vi "Datalog Aggregator.vi"(5 "LuaVIEW reference":T1) -> (15 "error out":errorcluster)   [LabVIEW 2012]
doc: "This plug-in is required by the \"datalogging\" runlevel. It sets up the buffer that aggregates data to be logged and periodically copies over the data from the in-memory tag buffers while applying logging algorithms."
uses:
  luaview/typedefs/t_LuaVIEW Reference.ctl
  typedefs/t_Datalog Aggregator States.ctl
  typedefs/t_DataLog Aggregate New Points Methods.ctl
  typedefs/t_DataLog Tag Info List Methods.ctl
  typedefs/t_DataLog Tag Buffers Methods.ctl
  luaview/typedefs/t_LuaVIEW Task State Methods.ctl
  typedefs/t_DataLog Aggregation Buffer Methods.ctl
  typedefs/t_DataLog Tag Hash Methods.ctl
  subvis/private/glb_DataLog Runtime Parameterisation.vi
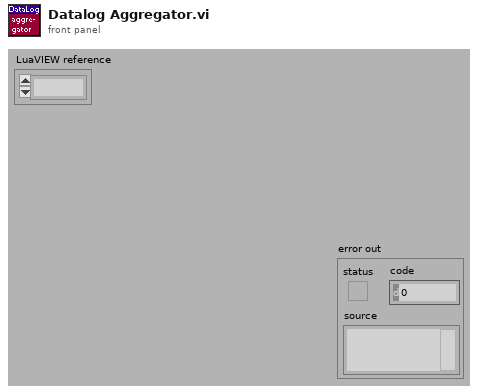
[diagram p1: front panel]
types:
  T1 = typedef "t_LuaVIEW Reference.ctl" = refnum<k1>
  T2 = typedef "t_Datalog Aggregator States.ctl" = enum16{"empty queue", "do aggregation", "undefine", "initialize", "init aggreg obj", "init undefine", "init active", "cleanup", "clean undefine", "clean buffers", "clean aggreg obj", "clean flush", "stop"}
  T3 = typedef "t_DataLog Aggregate New Points Methods.ctl" = enum16{"initialize", "aggregate", "cleanup"}
  T4 = typedef "t_DataLog Tag Info List Methods.ctl" = enum16{"initialize", "create", "create empty", "rename", "delete", "test tag", "get", "get by name", "get default", "get list", "get path", "get subsets", "set subsets", "set config", "set capacity", "#tags", "go live", "set unlocked", "set mirrored"}
  T5 = typedef "t_DataLog Tag Buffers Methods.ctl" = enum16{"initialize", "inert", "write", "read", "read oldest", "read last", "cleanup"}
  T6 = typedef "t_LuaVIEW Task State Methods.ctl" = enum16{"cleanup", "set initial", "set mode", "set active mode", "set error", "get task info", "get script info", "set signal", "clear signal", "test handled", "test delegated", "test signal", "handle signal", "delegate signal", "allow signal", "disallow signal", "disallow all", "signals?", "delegated signals?", "protection++", "protection--", "protection=0", "message", "next message", "pop message", "message available?", "force stop", "set swap preps", "apply swap preps"}
  T7 = typedef "t_DataLog Tag Hash Methods.ctl" = enum16{"initialize", "add tag", "index tag", "lookup", "#tags", "cleanup", "write recovery", "read recovery", "delete recovery"}
  T8 = typedef "t_DataLog Aggregation Buffer Methods.ctl" = enum16{"initialize", "write", "write special", "flush", "flush next", "flush next if", "setup recovery", "update recovery", "verify recovery", "dummy flush ", "cleanup"}
  T9 = typedef "t_DataLog Tag Config.ctl" = cluster{"name":string, "unit":string, "temporal":T10, "value":T11, "index":i32, "capacity":i32, "is meta?":bool, "mincapacity":i32, "deadband":dbl, "limit delay":dbl, "format":T12, "precision":u8, "undefine":bool, "update":bool, "update period":u16, "expression":string, "description":string, "logging algorithm":T13, "logging parameters":dbl[]}
  T10 = typedef "t_DataLog Temporal Types.ctl" = enum16{"set&hold", "sample", "event"}
  T11 = typedef "t_DataLog Value Types.ctl" = enum16{"number", "string"}
  T12 = typedef "t_DataLog Numerical Format.ctl" = enum8{"fractional", "exponential", "engineering"}
  T13 = typedef "t_DataLog Logging Algorithms.ctl" = enum16{"nothing", "changes", "everything", "every Nth", "time threshold", "value threshold + prior", "t or v threshold", "t or v threshold + prior"}
  T14 = typedef "t_DataLog Point.ctl" = cluster{"time":dbl, "value":dbl}
  T15 = typedef "t_LuaVIEW Task State Pane.ctl" = refnum<vi>
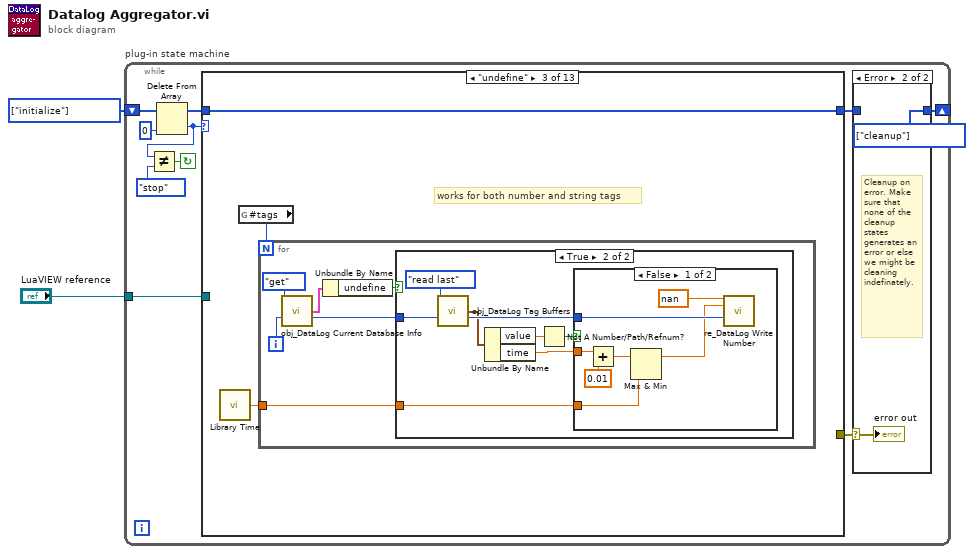
[diagram p0: block diagram]
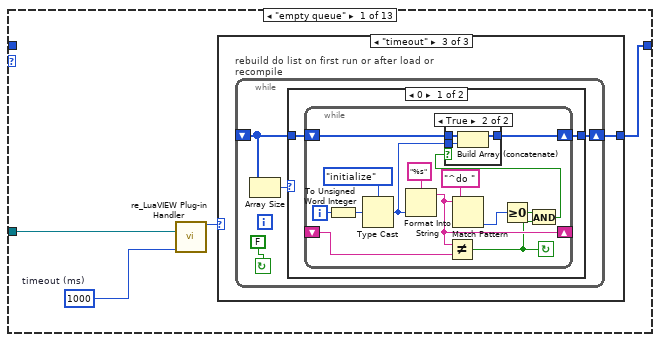
[diagram p3: hidden frame]
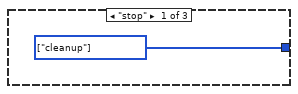
[diagram p4: hidden frame]
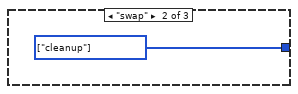
[diagram p5: hidden frame]
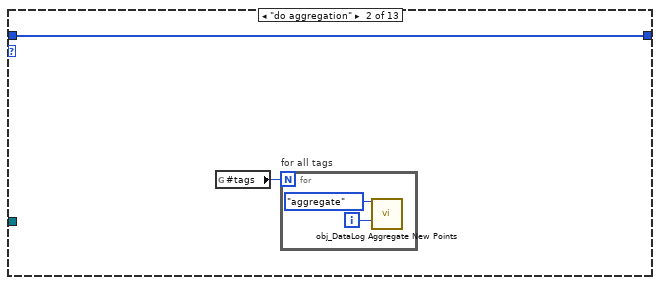
[diagram p8: hidden frame]
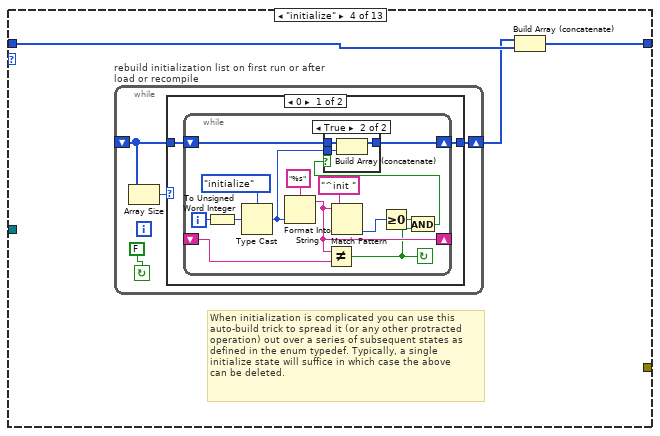
[diagram p11: hidden frame]
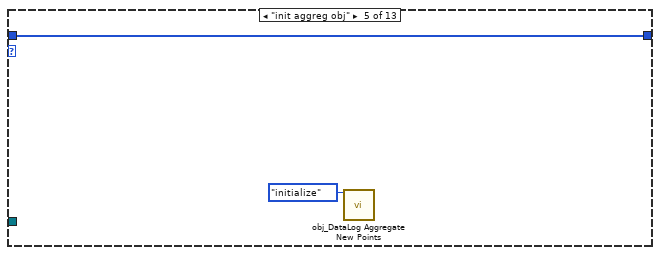
[diagram p14: hidden frame]
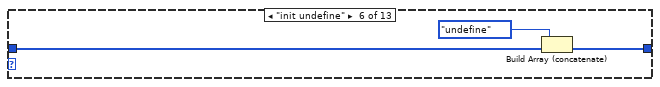
[diagram p15: hidden frame]
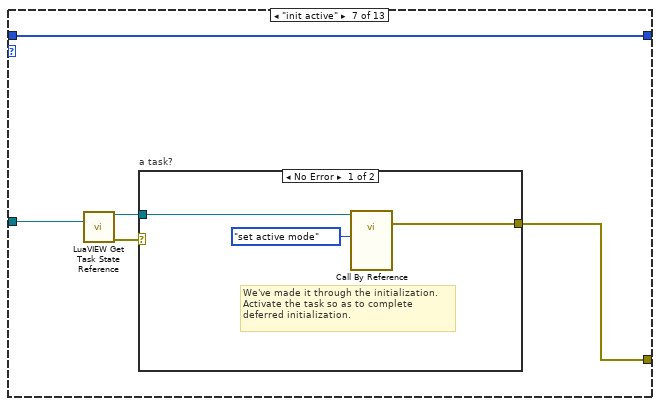
[diagram p16: hidden frame]
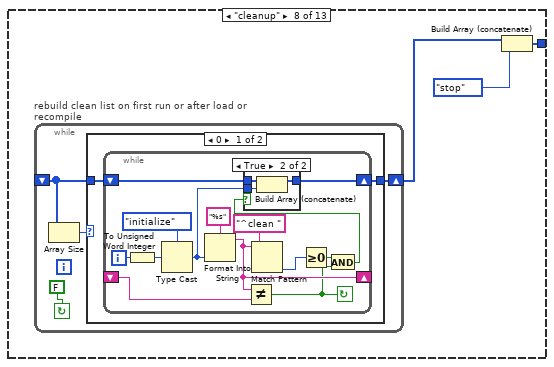
[diagram p18: hidden frame]
diagram:
  w2 = T2[] [enum."initialize"] items=["empty queue", "do aggregation", "undefine", "initialize", "init aggreg obj", "init undefine", "init active", "cleanup", "clean undefine", "clean buffers", "clean aggreg obj", "clean flush", "stop"] ("Array Constant")
  n1 = while "plug-in state machine" {
    shift-left: w2 -> [w10]
    shift-right: [w5] -> _
    tunnel: "LuaVIEW reference" -> [w7]
    stop <- w12 continue-if-true
    n2 = Delete From Array(array=w10, index=0) -> (deleted portion=w3:T2, array with subset deleted=w9:T2[])  [unwired: 1 in]
    n3 = Not Equal?(x=w3, y=t_Datalog_Aggregator_States."stop" ("states")) -> (x != y?=w12:bool)
    n4 = case "Case" shown="\"undefine\"" w3 {
      tunnel: [w19 w49 w54 w78 w105 w107 w113 w119 w146 w150 w152 w153 w159] -> w6
      tunnel: w9 -> [_ w49 w54 w77 w105 w108 w113 _ w147 w148 w152 w153 w159]
      tunnel: w7 -> [w17 _ _ _ _ _ w110 _ _ _ _ _ _]
      tunnel: [_ _ _ _ _ _ w112 _ _ _ _ _ _] -> w4
      frame "empty queue" {
        w16 = 1000  # timeout (ms)
        n5 = call "re_LuaVIEW Plug-in Handler.vi"("LuaVIEW reference"=w17, "timeout (ms)"=w16) -> ("handle"=w18:enum16{"timeout", "swap", "stop"})  [unwired: 13 in]
        n6 = case shown="\"timeout\"" w18 {
          tunnel: [w20 w21 w22] -> w19
          frame "stop" {
            w20 = T2[] [enum."cleanup"] items=["empty queue", "do aggregation", "undefine", "initialize", "init aggreg obj", "init undefine", "init active", "cleanup", "clean undefine", "clean buffers", "clean aggreg obj", "clean flush", "stop"] ("Array Constant")
          }
          frame "swap" {
            w21 = T2[] [enum."cleanup"] items=["empty queue", "do aggregation", "undefine", "initialize", "init aggreg obj", "init undefine", "init active", "cleanup", "clean undefine", "clean buffers", "clean aggreg obj", "clean flush", "stop"] ("Array Constant")
          }
          frame "timeout" {
            n7 = while "rebuild do list on first run or after load or recompile" {
              shift-left: _ -> [w25]
              shift-right: [w24] -> w22
              stop <- FALSE continue-if-true
              n8 = Array Size(array=w25) -> (size(s)=w26:i32)
              n9 = case shown="0" w26 {
                tunnel: [w27 w47] -> w24
                tunnel: w25 -> [w28 w47]
                frame 0 {
                  n10 = while {
                    shift-left: w28 -> [w38]
                    shift-right: [w36] -> w27
                    shift-left: _ -> [w39]
                    shift-right: [w35] -> _
                    i -> [w42]
                    stop <- w31 continue-if-true
                    n11 = To Unsigned Word Integer(number=w42) -> (unsigned 16bit integer=w40:u16)
                    n12 = Type Cast(type=t_Datalog_Aggregator_States."initialize" ("states"), x=w40) -> (*(type *) &x=w37:T2)
                    n13 = Format Into String(format string="%s" ("Format String"), w37) -> (resulting string=w35:string)  [unwired: 2 in, 1 out]
                    n14 = Not Equal?(x=w35, y=w39) -> (x != y?=w31:bool)
                    n15 = Match Pattern(string=w35, regular expression="^do ") -> (offset past match=w33:i32)  [unwired: 1 in, 3 out]
                    n16 = Greater Or Equal To 0?(x=w33) -> (x >= 0?=w32:bool)
                    n17 = And(x=w32, y=w31) -> (x .and. y?=w30:bool)
                    n18 = case shown="True" w30 {
                      tunnel: w38 -> [w43 w46]
                      tunnel: w37 -> [_ w45]
                      tunnel: [w43 w44] -> w36
                      frame False {
                      }
                      frame True {
                        n19 = Build Array (concatenate)(w46, w45) -> (w44:T2[])
                      }
                    }
                  }
                }
                frame Default {
                }
              }
            }
          }
        }
      }
      frame "do aggregation" {
        n20 = global read "glb_DataLog Runtime Parameterisation.vi" "#tags"() -> (w48:i32)
        n21 = for "for all tags" {
          N: w48 -> [_]
          i -> [w51]
          n22 = call "obj_DataLog Aggregate New Points.vi"("method"=t_DataLog_Aggregate_New_Points_Methods."aggregate", "tag index in"=w51) -> ()  [unwired: 13 in, 1 out]
        }
      }
      frame "undefine" {
        # "works for both number and string tags"
        n23 = call "Library Time.vi"() -> ("time"=w52:dbl)  [unwired: 1 in]
        n24 = global read "glb_DataLog Runtime Parameterisation.vi" "#tags"() -> (w53:i32)
        n25 = for {
          N: w53 -> [_]
          tunnel: w52 -> [w55]
          i -> [w60]
          n26 = call "obj_DataLog Current Database Info.vi"("method"=t_DataLog_Tag_Info_List_Methods."get", "tag index/change#"=w60) -> ("tag config out"=w57:T9, "dup tag index"=w59:i32)  [unwired: 7 in, 5 out]
          n27 = Unbundle By Name(w57) -> ("undefine"=w56:bool)
          n28 = case shown="True" w56 {
            tunnel: w59 -> [_ w68]
            tunnel: w55 -> [_ w61]
            frame False {
            }
            frame True {
              n29 = call "obj_DataLog Tag Buffers.vi"("method"=t_DataLog_Tag_Buffers_Methods."read last", "tag index"=w68) -> ("point out"=w62:T14, "tag index dup"=w65:i32)  [unwired: 9 in, 3 out]
              n30 = Unbundle By Name(w62) -> ("value"=w66:dbl, "time"=w63:dbl)
              n31 = Not A Number/Path/Refnum?(number/path/refnum=w66) -> (NaN/Path/Refnum?=w64:bool)
              n32 = case shown="False" w64 {
                tunnel: w65 -> [w75 _]
                tunnel: w63 -> [w74 _]
                tunnel: w61 -> [w71 _]
                frame False {
                  n33 = Add(x=w74, y=0.01) -> (x+y=w72:dbl)
                  n34 = Max & Min(x=w72, y=w71) -> (max(x,y)=w69:dbl)  [unwired: 1 out]
                  n35 = call "re_DataLog Write Number.vi"("number"=nan ("value"), "time (current)"=w69, "tag index in (use tag)"=w75) -> ()  [unwired: 11 in, 2 out]
                }
                frame True {
                }
              }
            }
          }
        }
      }
      frame "initialize" {
        # "When initialization is complicated you can use this\nauto-build trick to spread it (or any other protracted\noperation) out over a series of subsequent states as\ndefined in the enum typedef. Typically, a single\ninitialize state will suffice in which case the above\ncan be deleted."
        n36 = while "rebuild initialization list on first run or after load or recompile" {
          shift-left: _ -> [w81]
          shift-right: [w80] -> w76
          stop <- FALSE continue-if-true
          n37 = Array Size(array=w81) -> (size(s)=w82:i32)
          n38 = case shown="0" w82 {
            tunnel: [w83 w103] -> w80
            tunnel: w81 -> [w84 w103]
            frame 0 {
              n39 = while {
                shift-left: w84 -> [w93]
                shift-right: [w91] -> w83
                shift-left: _ -> [w95]
                shift-right: [w90] -> _
                i -> [w98]
                stop <- w86 continue-if-true
                n40 = To Unsigned Word Integer(number=w98) -> (unsigned 16bit integer=w96:u16)
                n41 = Type Cast(type=t_Datalog_Aggregator_States."initialize" ("states"), x=w96) -> (*(type *) &x=w92:T2)
                n42 = Format Into String(format string="%s" ("Format String"), w92) -> (resulting string=w90:string)  [unwired: 2 in, 1 out]
                n43 = Not Equal?(x=w90, y=w95) -> (x != y?=w86:bool)
                n44 = Match Pattern(string=w90, regular expression="^init ") -> (offset past match=w88:i32)  [unwired: 1 in, 3 out]
                n45 = Greater Or Equal To 0?(x=w88) -> (x >= 0?=w87:bool)
                n46 = And(x=w87, y=w86) -> (x .and. y?=w85:bool)
                n47 = case shown="True" w85 {
                  tunnel: w93 -> [w99 w102]
                  tunnel: w92 -> [_ w101]
                  tunnel: [w99 w100] -> w91
                  frame False {
                  }
                  frame True {
                    n48 = Build Array (concatenate)(w102, w101) -> (w100:T2[])
                  }
                }
              }
            }
            frame Default {
            }
          }
        }
        n49 = Build Array (concatenate)(w76, w77) -> (w78:T2[])
      }
      frame "init aggreg obj" {
        n50 = call "obj_DataLog Aggregate New Points.vi"("method"=t_DataLog_Aggregate_New_Points_Methods."initialize") -> ()  [unwired: 14 in, 1 out]
      }
      frame "init undefine" {
        n51 = Build Array (concatenate)(t_Datalog_Aggregator_States."undefine" ("states"), w108) -> (w107:T2[])
      }
      frame "init active" {
        n52 = call "LuaVIEW Get Task State Reference.vi"("LuaVIEW reference in"=w110) -> ("task state reference"=w109:T15, "error out"=w111:errorcluster)  [unwired: 12 in, 1 out]
        n53 = case "a task?" shown="No Error" w111 {
          tunnel: w109 -> [w115 _]
          tunnel: [w114 _] -> w112
          frame No Error {
            # "We've made it through the initialization.\nActivate the task so as to complete\ndeferred initialization."
            n54 = call-by-ref "?"(reference=w115, "method"=t_LuaVIEW_Task_State_Methods."set active mode") -> (error out=w114:errorcluster)  [unwired: 11 in, 6 out]
          }
          frame Error {
          }
        }
      }
      frame "cleanup" {
        n55 = while "rebuild clean list on first run or after load or recompile" {
          shift-left: _ -> [w122]
          shift-right: [w121] -> w117
          stop <- FALSE continue-if-true
          n56 = Array Size(array=w122) -> (size(s)=w123:i32)
          n57 = case shown="0" w123 {
            tunnel: [w124 w144] -> w121
            tunnel: w122 -> [w125 w144]
            frame 0 {
              n58 = while {
                shift-left: w125 -> [w135]
                shift-right: [w133] -> w124
                shift-left: _ -> [w136]
                shift-right: [w132] -> _
                i -> [w139]
                stop <- w128 continue-if-true
                n59 = To Unsigned Word Integer(number=w139) -> (unsigned 16bit integer=w137:u16)
                n60 = Type Cast(type=t_Datalog_Aggregator_States."initialize" ("states"), x=w137) -> (*(type *) &x=w134:T2)
                n61 = Format Into String(format string="%s" ("Format String"), w134) -> (resulting string=w132:string)  [unwired: 2 in, 1 out]
                n62 = Not Equal?(x=w132, y=w136) -> (x != y?=w128:bool)
                n63 = Match Pattern(string=w132, regular expression="^clean ") -> (offset past match=w130:i32)  [unwired: 1 in, 3 out]
                n64 = Greater Or Equal To 0?(x=w130) -> (x >= 0?=w129:bool)
                n65 = And(x=w129, y=w128) -> (x .and. y?=w127:bool)
                n66 = case shown="True" w127 {
                  tunnel: w135 -> [w140 w143]
                  tunnel: w134 -> [_ w142]
                  tunnel: [w140 w141] -> w133
                  frame False {
                  }
                  frame True {
                    n67 = Build Array (concatenate)(w143, w142) -> (w141:T2[])
                  }
                }
              }
            }
            frame Default {
            }
          }
        }
        n68 = Build Array (concatenate)(w117, t_Datalog_Aggregator_States."stop" ("states")) -> (w119:T2[])
      }
      frame "clean undefine" {
        n69 = Build Array (concatenate)(t_Datalog_Aggregator_States."undefine" ("states"), w147) -> (w146:T2[])
      }
      frame "clean buffers" {
        n70 = Build Array (concatenate)(t_Datalog_Aggregator_States."do aggregation" ("states"), w148) -> (w150:T2[])
      }
      frame "clean aggreg obj" {
        n71 = call "obj_DataLog Aggregate New Points.vi"("method"=t_DataLog_Aggregate_New_Points_Methods."cleanup") -> ()  [unwired: 14 in, 1 out]
      }
      frame "clean flush" {
        # "Flush the remaining unflushed data in the aggregation buffer. Delete the hash recovery to signal that there is nothing left that needs recovering."
        n72 = while "flush all unflushed tags" {
          tunnel: [t_DataLog_Tag_Hash_Methods."delete recovery" ("method")] -> w154
          stop <- w155 continue-if-true
          n73 = call "obj_DataLog Aggregation Buffer.vi"("method"=t_DataLog_Aggregation_Buffer_Methods."flush next") -> ("flush needed?"=w155:bool, "error out"=w156:errorcluster)  [unwired: 13 in]
          n74 = call "ClientSrv Log Server Error.vi"("error (use message)"=w156) -> ()  [unwired: 15 in]
        }
        n75 = call "obj_DataLog Tag Hash.vi"("method"=w154) -> ()  [unwired: 11 in, 4 out]
      }
      frame "stop" {
        # "The very last state."
      }
    }
    n76 = case shown="Error" w4 {
      selector: w4 -> [_ w14]
      tunnel: w6 -> [w13 _]
      tunnel: [w13 w15] -> w5
      frame No Error {
      }
      frame Error {
        w15 = T2[] [enum."cleanup"] items=["empty queue", "do aggregation", "undefine", "initialize", "init aggreg obj", "init undefine", "init active", "cleanup", "clean undefine", "clean buffers", "clean aggreg obj", "clean flush", "stop"] ("Array Constant")
        # "Cleanup on error. Make sure that none of the cleanup states generates an error or else we might be cleaning indefinately."
        "error out" <- w14
      }
    }
  }
